vi "StatusBooleanEdgeTrigger.vi"(11 "Boolean Input":bool) -> (2 "Falling Edge":bool, 3 "Rising Edge":bool)   [LabVIEW 2020]
doc: "This VI is used to detect rising and falling edges of the Boolean Input. \"Rising Edge\" is TRUE if Boolean Input is TRUE and was previously FALSE. \"Falling Edge\" is TRUE if Boolean Input is FALSE and was previously TRUE. This VI is intended to be used in loops to aid in user input polling."
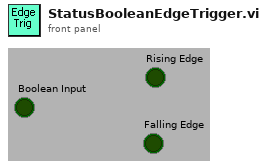
[diagram p1: front panel]
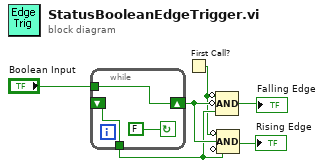
[diagram p0: block diagram]
diagram:
  n1 = while {
    tunnel: [w8] -> w5
    tunnel: "Boolean Input" -> [w9]
    shift-left: _ -> [w8]
    shift-right: [w9] -> w6
    stop <- FALSE continue-if-true
  }
  n2 = First Call?() -> (First Call?: T/F=w1:bool)
  n3 = Compound Arithmetic op=AND(invert w1, invert w6, w5) -> (→"Falling Edge":bool)
  n4 = Compound Arithmetic op=AND(invert w1, w6, invert w5) -> (→"Rising Edge":bool)
